vi "(SubVI) x range set.vi"(9 "lower limit":dbl, 10 "x":dbl, 11 "upper limit":dbl) -> (3 "Boolean":bool)   [LabVIEW 2016]
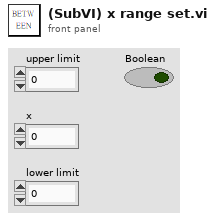
[diagram p1: front panel]
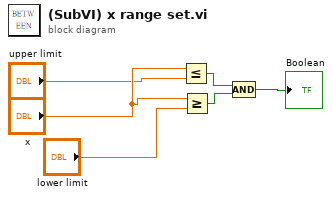
[diagram p0: block diagram]
diagram:
  n1 = Less Or Equal?(x="x", y="upper limit") -> (x <= y?=w1:bool)
  n2 = Greater Or Equal?(x="x", y="lower limit") -> (x >= y?=w2:bool)
  n3 = Compound Arithmetic op=AND(w1, w2) -> (→"Boolean":bool)
